vi "Set MFC Flows.vi"(8 "error in":errorcluster, 10 "Setpoints":sgl[](array[numeric]), 11 "CRDS in":refnum<class "CRDS.lvclass">) -> (0 "error out":errorcluster, 3 "CRDS out":refnum<class "CRDS.lvclass">)   [LabVIEW 2011, in "CRDS.lvclass"]
uses:
  CRDS.lvclass
  Reusable/Serial IO/Alicat/AlicatCommBank/AlicatCommBank.lvclass
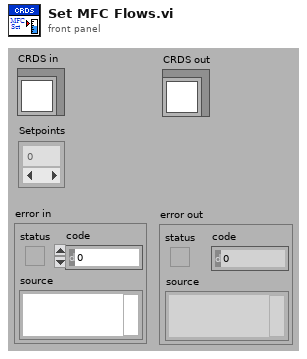
[diagram p1: front panel]
types:
  T1 = cluster{"YAG Ctr":refnum<k21>, "Diode Ctr":refnum<k21>, "Gated Ctr":refnum<k21>, "LF AI":refnum<k21>, "HF AI":refnum<k21>, "valveIn":refnum<k21>, "valveOut":refnum<k21>}
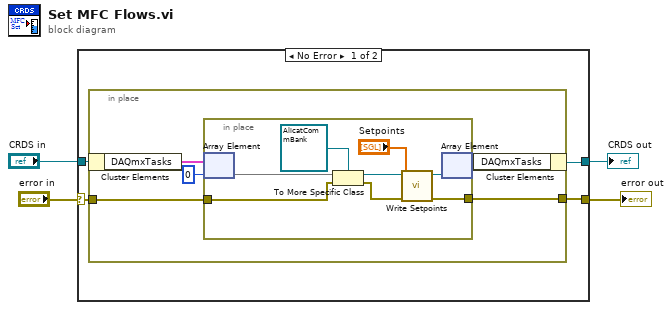
[diagram p0: block diagram]
diagram:
  n1 = case shown="No Error" "error in" {
    selector: "error in" -> [w6 w22]
    tunnel: "CRDS in" -> [w8 w23]
    tunnel: [w7 w23] -> w3
    tunnel: [w5 w22] -> w1
    frame No Error {
      n2 = in-place {
        in-place-border: w6 -> [w10]
        in-place-border: [w9] -> w5
        n3 = in-place-cluster #1(w8) -> ("DAQmxTasks"=w13:T1)
        n4 = in-place {
          in-place-border: w10 -> [w17]
          in-place-border: [w14] -> w9
          n5 = in-place-array #2(w13, 0) -> (w19)
          n6 = To More Specific Class(target class=refnum<class "AlicatCommBank.lvclass"> refnum ("AlicatCommBank.lvclass"), reference=w19, error in=w17) -> (specific class reference=w20:refnum<class "AlicatCommBank.lvclass">, error out=w16:errorcluster)
          n7 = call-dynamic "Write Setpoints.vi"("error in"=w16, "Setpoints"="Setpoints", "AlicatCommBank in"=w20) -> ("error out"=w14:errorcluster, "AlicatCommBank out"=w15:refnum<class "AlicatCommBank.lvclass">)  [unwired: 7 in]
          n8 = in-place-array #2(w15) -> (w12)  [unwired: 1 out]
        }
        n9 = in-place-cluster #1("DAQmxTasks"=w12) -> (w7:refnum<class "CRDS.lvclass">)
      }
    }
    frame Error {
    }
  }
  "error out" <- w1
  "CRDS out" <- w3
